vi "Extract Numbers.vi"(0 "Strimg[]":string[](array[string])) -> (1 "I32[]":i32[](array[numeric]), 2 "Sgl[]":dbl[](array[numeric]) format="%.2f")   [LabVIEW 2011]
doc: "Finds all numbers in the given string and puts them into an array as single-precision numbers. All of the following formats are recognized:\n123 1.23 1.23e2 1.23E2\nNo spaces or other characters may appear within the number, but any characters may appear before or after the number."
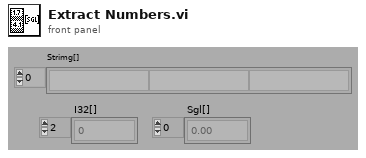
[diagram p1: front panel]
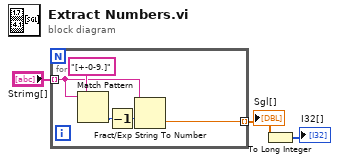
[diagram p0: block diagram]
diagram:
  n1 = for {
    tunnel: [w6] -> w2 mode=indexing
    tunnel: "Strimg[]" -> [w5] mode=indexing
    n2 = Match Pattern(string=w5, regular expression="[+-0-9.]") -> (offset past match=w7:i32)  [unwired: 1 in, 3 out]
    n3 = Decrement(x=w7) -> (x-1=w4:i32)
    n4 = Fract/Exp String To Number(string=w5, offset=w4) -> (number=w6:dbl)  [unwired: 2 in, 1 out]
  }
  "Sgl[]" <- w2
  n5 = To Long Integer(number=w2) -> (32bit integer=→"I32[]":i32[])
